vi "Read_Timestamp_from_TDMS.vi"(8 "error in (no error)":errorcluster, 11 "TDMS File path":path) -> (0 "error out":errorcluster, 2 "Number of timestamps":i32, 3 "relative timestamp (s)":dbl[](array[numeric]))   [LabVIEW 2020]
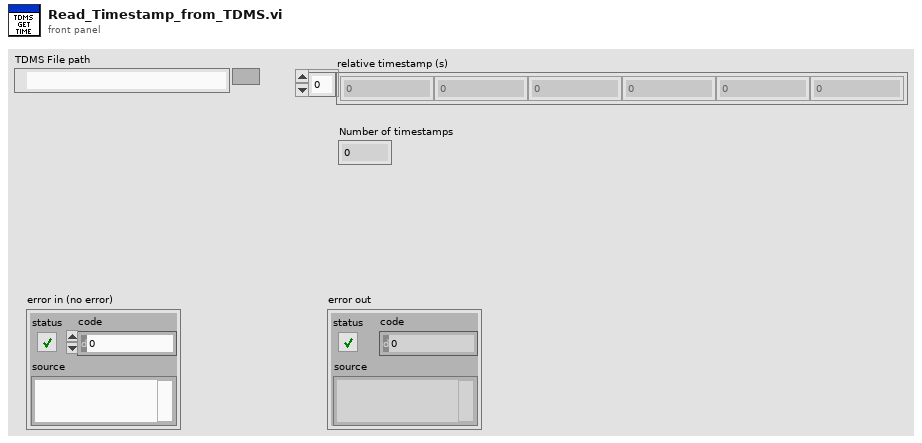
[diagram p1: front panel]
types:
  T1 = enum16{"open", "open or create", "create or replace", "create", "open (read-only)"}
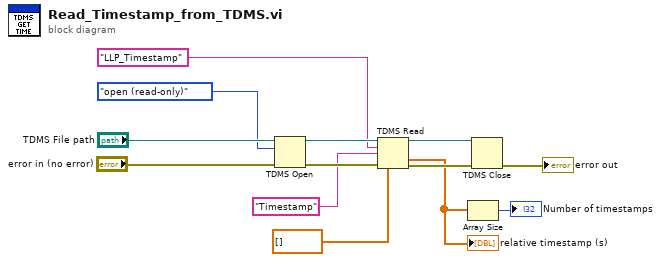
[diagram p0: block diagram]
diagram:
  n1 = TDMS Open(8:"error in (no error)", 10:T1."open (read-only)" ("operation (0:open)"), 11:"TDMS File path") -> (0:w9:errorcluster, 3:w10:refnum<k34>)  [unwired: 4 in]
  n2 = TDMS Read(0:w10, 5:"LLP_Timestamp" ("Save to Group"), 7:"Timestamp" ("channel name"), 11:w9, 12:dbl[] []) -> (4:w5:refnum<k34>, 10:w2:dbl[], 15:w4:errorcluster)  [unwired: 3 in, 3 out]
  "relative timestamp (s)" <- w2
  n3 = Array Size(array=w2) -> (size(s)=→"Number of timestamps":i32)
  n4 = TDMS Close(8:w4, 11:w5) -> (0:→"error out":errorcluster)  [unwired: 1 out]
